vi "dfd_Get Quantized MRate Coef.vi"(7 "coef wl":i16, 8 "L":i32, 9 "scale type":T3=enum."Time Domain 1-Norm", 10 "scale by Power of 2?":bool, 11 "h":dbl[](array[numeric])) -> (0 "coef quantizer":T1={"source"=0, "wl"=16, "iwl"=1, "overflow mode"=enum."Wrap", "rounding mode"=enum."Truncation", "signed?"=TRUE} {"source" items=["Coefficients a/k"=0, "Coefficients b/v"=7, "Input"=1, "Output"=2, "Multiplicand"=3, "Product"=4, "Sum"=5, "Delay"=6]}, 3 "h (I32)":i32[](array[numeric]))   [LabVIEW 2017, in "NI_DigFilter_FXP.lvlib"]
uses:
  <vilib>/addons/Digital Filter Design/NI_DigFilter_FXP.lvlib
  <vilib>/addons/Digital Filter Design/_Objects.llb/DFD Coef Norm Type.ctl
  <vilib>/addons/Digital Filter Design/_Objects.llb/DFD Quantization Settings.ctl
  <vilib>/addons/Digital Filter Design/_Objects.llb/DFD Quantization Sources.ctl
  <vilib>/addons/Digital Filter Design/NI_DigFilterLicensed.lvlib
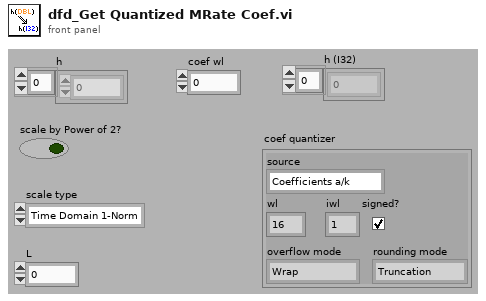
[diagram p1: front panel]
types:
  T1 = typedef "NI_DigFilterLicensed.lvlib/DFD Quantization Settings.ctl" = cluster{"source":T2, "wl":i16, "iwl":i16, "overflow mode":enum16{"Saturation", "Wrap"}, "rounding mode":enum16{"Nearest", "Truncation"}, "signed?":bool}
  T2 = typedef "NI_DigFilterLicensed.lvlib/DFD Quantization Sources.ctl" = u16
  T3 = typedef "NI_DigFilterLicensed.lvlib/DFD Coef Norm Type.ctl" = enum16{"No Norm", "Time Domain 1-Norm", "Time Domain 2-Norm", "Time Domain Inf-Norm"}
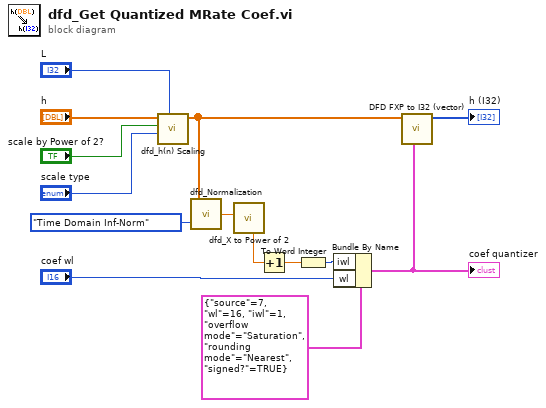
[diagram p0: block diagram]
diagram:
  n1 = call <vilib>:"dfd_h(n) Scaling.vi"("L"="L", "scale type"="scale type", "scale by Power of 2?"="scale by Power of 2?", "h(n)"="h") -> ("scaled  h(n)"=w7:dbl[])  [unwired: 7 out]
  n2 = call <vilib>:"dfd_Normalization.vi"("scale type"=DFD_Coef_Norm_Type."Time Domain Inf-Norm", "h(n)"=w7) -> ("norm"=w5:dbl)
  n3 = call <vilib>:"dfd_X to Power of 2.vi"("x"=w5) -> ("n"=w4:dbl)  [unwired: 10 out]
  n4 = Increment(x=w4) -> (x+1=w3:dbl)
  n5 = To Word Integer(number=w3) -> (16bit integer=w2:i16)
  n6 = Bundle By Name(cluster=T1 {"source"=7, "wl"=16, "iwl"=1, "overflow mode"=enum."Saturation", "rounding mode"=enum."Nearest", "signed?"=TRUE} ("quantization settings"), "iwl"=w2, "wl"="coef wl") -> (w12:T1)
  "coef quantizer" <- w12
  n7 = call <vilib>:"DFD FXP to I32 (vector).vi"("quantization settings"=w12, "FXP values"=w7) -> ("I32 values"=→"h (I32)":i32[])  [unwired: 1 in, 8 out]
